vi "chart series set trendline r squared.vi"(8 "error in (no error)":errorcluster, 11 "series":u32) -> (0 "error out":errorcluster)   [LabVIEW 8.6]
doc: "void chart_series_set_trendline_r_squared(lxw_chart_series series);"
uses:
  pending_lvxlsxwriter/xlsxwriter.dll
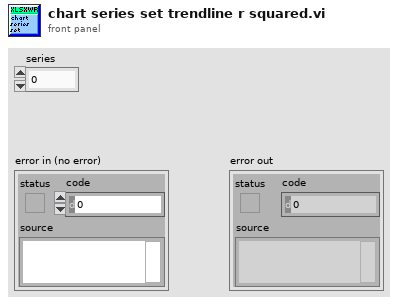
[diagram p1: front panel]
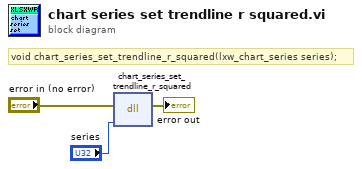
[diagram p0: block diagram]
diagram:
  # "void chart_series_set_trendline_r_squared(lxw_chart_series series);"
  n1 = dll-call lib="C:/Users/WDAGUtilityAccount/Desktop/pending_lvxlsxwriter/xlsxwriter.*" fn="chart_series_set_trendline_r_squared"(error in="error in (no error)", "series"="series") -> (error out=→"error out":errorcluster)  [unwired: 4 in, 1 out]
